vi "Close.vi"(8 "error in (no error)":errorcluster, 11 "Laser Diode Controller in":refnum<class "KLD101.lvclass">) -> (0 "error out":errorcluster)   [LabVIEW 2016, in "Laser Diode Controller.lvlib" / "KLD101.lvclass"]
uses:
  KLD101.lvclass
  KLD101.lvclass/KLD101.ctl
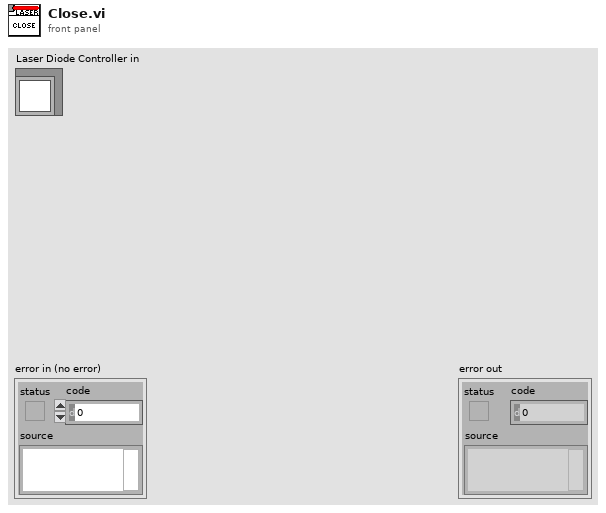
[diagram p1: front panel]
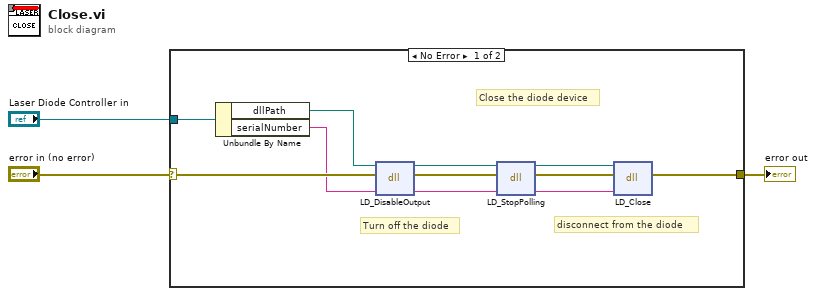
[diagram p0: block diagram]
diagram:
  n1 = case shown="No Error" "error in (no error)" {
    selector: "error in (no error)" -> [w13 w15]
    tunnel: [w12 w15] -> w2
    tunnel: "Laser Diode Controller in" -> [w14 _]
    frame No Error {
      # "disconnect from the diode"
      # "Turn off the diode"
      # "Close the diode device"
      n2 = Unbundle By Name(w14) -> ("dllPath"=w6:path, "serialNumber"=w11:string)
      n3 = dll-call lib="C:/IDEXX Software/Collimation/data/Thorlabs.MotionControl.KCube.LaserDiode.dll" fn="LD_DisableOutput"(path in=w6, error in=w13, "serialNumber"=w11) -> (path out=w5:path, error out=w8:errorcluster, "serialNumber"=w10:string)  [unwired: 2 in]
      n4 = dll-call lib="C:/IDEXX Software/Collimation/data/Thorlabs.MotionControl.KCube.LaserDiode.dll" fn="LD_StopPolling"(path in=w5, error in=w8, "serialNumber"=w10) -> (path out=w4:path, error out=w7:errorcluster, "serialNumber"=w9:string)  [unwired: 2 in]
      n5 = dll-call lib="C:/IDEXX Software/Collimation/data/Thorlabs.MotionControl.KCube.LaserDiode.dll" fn="LD_Close"(path in=w4, error in=w7, "serialNumber"=w9) -> (error out=w12:errorcluster)  [unwired: 3 in, 1 out]
    }
    frame Error {
    }
  }
  "error out" <- w2
